vi "ConvertDateFormat.vi"(11 "DataIn":string[][](array[string])=[["Admin", "0", "Admin", "Administrator", "123456", "1", "5", "0", "2018/02/01", "14:05:42"], ["Supervisor", "1", "Supervisor", "Production", "123456", "1", "5", "0", "2018/02/01", "14:05:42"], ["Operator", "2", "Operator", "Operator", "123456", "1", "5", "0", "2018/02/01", "14:05:42"]]) -> (3 "DataOut":string[][](array[string]))   [LabVIEW 2015]
uses:
  System Settings/Modules/LV2GActions.ctl
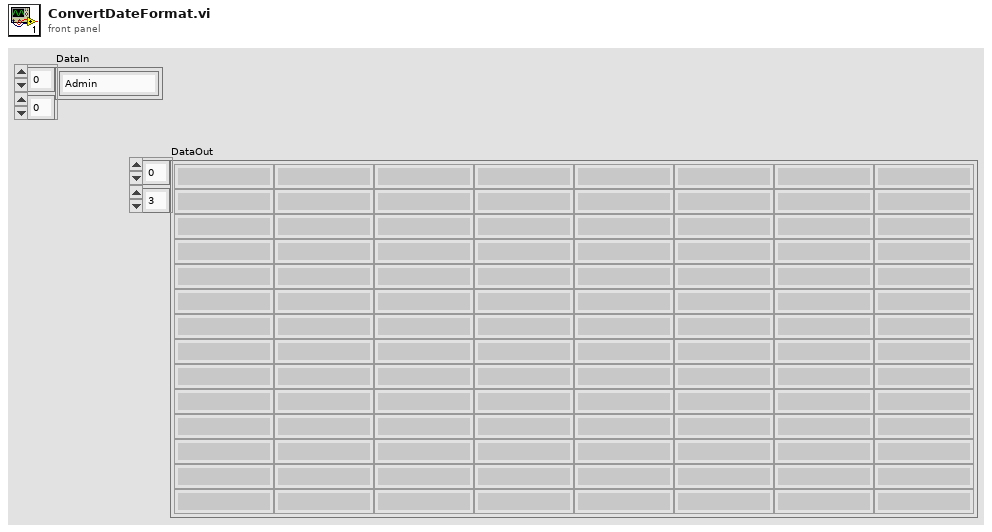
[diagram p1: front panel]
types:
  T1 = typedef "LV2GActions.ctl" = enum16{"Read", "Write", "Current", "Update", "UpdateSystemSettings", "UpdateModel"}
  T2 = cluster{"UserName":string, "Group Level":u16, "Theme":u16, "Software Type":u16, "System Language":u16, "Master":bool, "Recipe":string, "Batch":string, "Simulate":bool, "Trigger Activation":u16, "DateFormat":u16, "HardwareTest":bool}
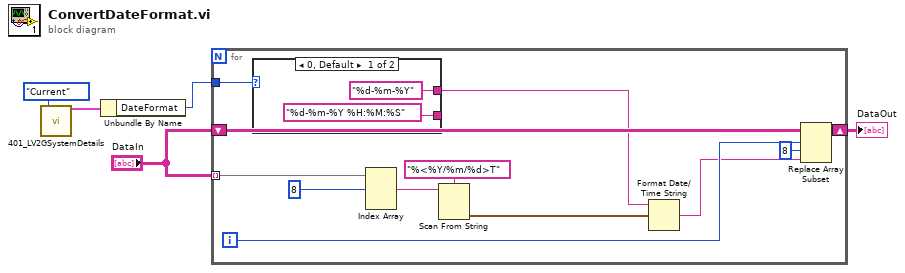
[diagram p0: block diagram]
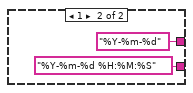
[diagram p2: hidden frame]
diagram:
  n1 = call "401_LV2GSystemDetails.vi"("R/W/C"=LV2GActions."Current") -> ("DataOut"=w5:T2)  [unwired: 17 in, 1 out]
  n2 = Unbundle By Name(w5) -> ("DateFormat"=w3:u16)
  n3 = for {
    shift-right: [w11] -> w1
    shift-left: "DataIn" -> [w14]
    tunnel: "DataIn" -> [w17] mode=indexing
    tunnel: w3 -> [w6]
    i -> [w9]
    n4 = case shown="0, Default" w6 {
      tunnel: ["%d-%m-%Y %H:%M:%S" ("time format string (%c)") "%Y-%m-%d %H:%M:%S" ("time format string (%c)")] -> _
      tunnel: ["%d-%m-%Y" ("time format string (%c)") "%Y-%m-%d" ("time format string (%c)")] -> w7
      frame 0, Default {
      }
      frame 1 {
      }
    }
    n5 = Index Array(array=w17, index #1=8 ("index")) -> (element #1=w15:string)  [unwired: 2 in, 2 out]
    n6 = Scan From String(format string="%<%Y/%m/%d>T" ("time format string (%c)"), input string=w15) -> (output 1=w12:timestamp)  [unwired: 3 in, 3 out]
    n7 = Format Date/Time String(time format string (%c)=w7, seconds (now)=w12) -> (date/time string=w8:string)  [unwired: 1 in]
    n8 = Replace Array Subset(array=w14, new element=w8, index (row)=w9, index (col)=8 ("disabled index (col)")) -> (w11:string[][])
  }
  "DataOut" <- w1
